vi "GV_Repos.vi"() -> ()   [LabVIEW 2020, in "WSsupport.lvlib"]
uses:
  WSsupport.lvlib
  Packages/Repo_class/Repo.lvclass
panel:
  in  "Repos":refnum<class "Repo.lvclass">[](array[class])
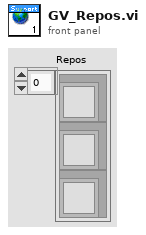
[diagram p1: front panel]
diagram:
